vi "Stream_UpdateInfo.vi"(8 "error in (no error)":errorcluster, 9 "Device":string, 10 "SendEventRef":T1, 11 "streams in":variant) -> (0 "error out":errorcluster, 1 "block number":i32, 3 "streams out":variant)   [LabVIEW 2017, in "FileManager.lvlib"]
uses:
  <vilib>/addons/InsightCM/Devices/Shared/Common/FileManager/FileManager.lvlib
  <vilib>/addons/InsightCM/Devices/Shared/Common/FileManager/controls/SendEventRefRoutedMessage.ctl
  <vilib>/addons/InsightCM/Devices/Shared/Common/DataEvent/controls/EventReference.ctl
  <vilib>/addons/InsightCM/Devices/Shared/Common/DataEvent/controls/Event.ctl
  <vilib>/addons/InsightCM/MessageBus/Base/controls/DataEvent.ctl
  <vilib>/addons/InsightCM/MessageBus/Base/controls/KeyValuePair.ctl
  <vilib>/addons/InsightCM/Devices/Shared/Common/DataEvent/controls/DataSet.ctl
  <vilib>/addons/InsightCM/MessageBus/Base/controls/DataSetMetadata.ctl
  <vilib>/addons/InsightCM/MessageBus/Base/controls/TrendPoint.ctl
  <vilib>/addons/InsightCM/MessageBus/Base/controls/TrendAlarmUpdate.ctl
  <vilib>/addons/InsightCM/MessageBus/Base/controls/TrendAlarmTransition.ctl
  <vilib>/addons/InsightCM/Devices/Shared/Common/FileManager/controls/StreamState.ctl
  <vilib>/addons/InsightCM/Devices/Shared/Common/DataEvent/DataEvent.lvlib
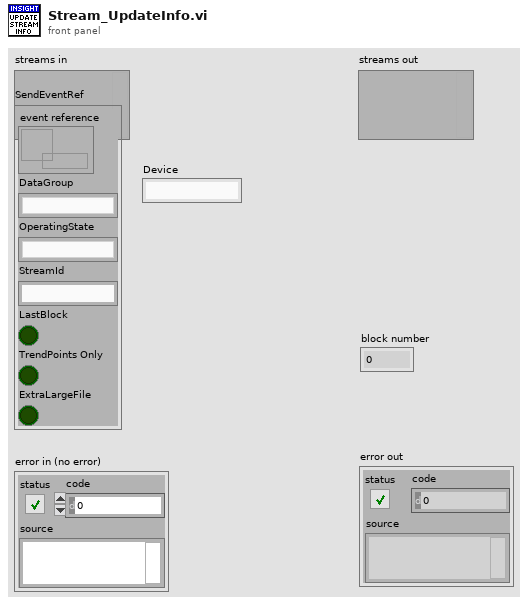
[diagram p1: front panel]
types:
  T1 = typedef "FileManager.lvlib/SendEventRefRoutedMessage.ctl" = cluster{"event reference":T2, "DataGroup":string, "OperatingState":string, "StreamId":string, "LastBlock":bool, "TrendPoints Only":bool, "ExtraLargeFile":bool}
  T2 = typedef "DataEvent.lvlib/EventReference.ctl" = refnum<data-value>
  T3 = typedef "FileManager.lvlib/StreamState.ctl" = cluster{"DataGroup":string, "Stream Id":string, "LastBlock":bool, "TotalBlocks":i32, "BlocksSent":i32, "Device":string}
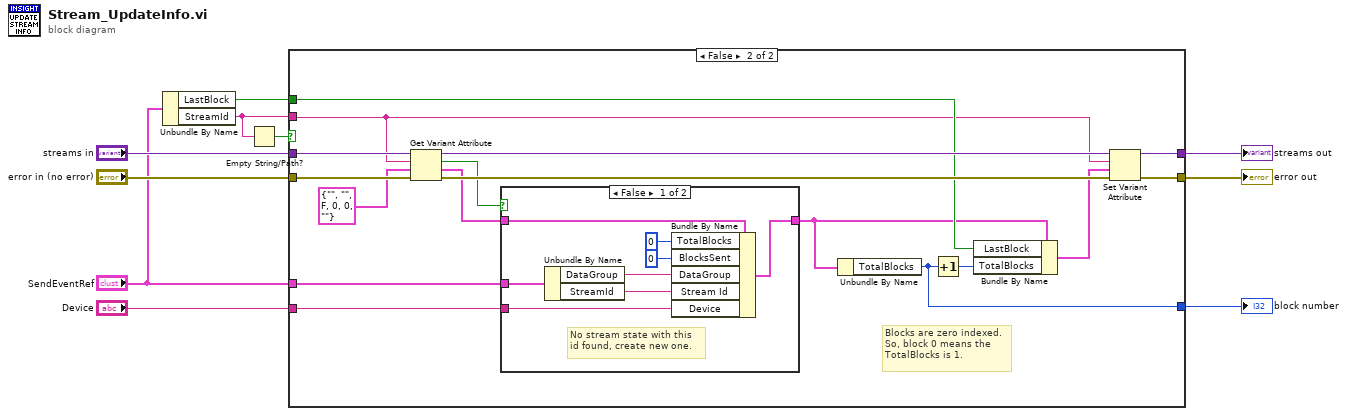
[diagram p0: block diagram]
diagram:
  n1 = Unbundle By Name("SendEventRef") -> ("LastBlock"=w4:bool, "StreamId"=w3:string)
  n2 = Empty String/Path?(string/path=w3) -> (empty?=w2:bool)
  n3 = case shown="False" w2 {
    tunnel: "streams in" -> [w12 w27]
    tunnel: [w12 w26] -> w9
    tunnel: [w11 w25] -> w8
    tunnel: "error in (no error)" -> [w11 w24]
    tunnel: [_ w23] -> w6
    tunnel: "SendEventRef" -> [_ w22]
    tunnel: w4 -> [_ w21]
    tunnel: w3 -> [_ w14]
    tunnel: "Device" -> [_ w13]
    frame True {
      # "If StreamId is empty, this is not a stream"
    }
    frame False {
      # "Blocks are zero indexed.\nSo, block 0 means the\nTotalBlocks is 1."
      n4 = Get Variant Attribute(Variant=w27, name=w14, default value (empty Variant)=T3 {"DataGroup"="", "Stream Id"="", "LastBlock"=FALSE, "TotalBlocks"=0, "BlocksSent"=0, "Device"=""} ("Stream"), error in=w24) -> (duplicate Variant=w28:variant, found=w17:bool, value=w15:T3, error out=w29:errorcluster)
      n5 = case shown="False" w17 {
        tunnel: w15 -> [w34 w38]
        tunnel: w22 -> [w37 _]
        tunnel: [w33 w38] -> w20
        tunnel: w13 -> [w30 _]
        frame False {
          # "No stream state with this \nid found, create new one."
          n6 = Unbundle By Name(w37) -> ("DataGroup"=w32:string, "StreamId"=w31:string)
          n7 = Bundle By Name(cluster=w34, "TotalBlocks"=0, "BlocksSent"=0, "DataGroup"=w32, "Stream Id"=w31, "Device"=w30) -> (w33:T3)
        }
        frame True {
        }
      }
      n8 = Unbundle By Name(w20) -> ("TotalBlocks"=w23:i32)
      n9 = Increment(x=w23) -> (x+1=w19:i32)
      n10 = Bundle By Name(cluster=w20, "LastBlock"=w21, "TotalBlocks"=w19) -> (w18:T3)
      n11 = Set Variant Attribute(Variant=w28, name=w14, value=w18, error in=w29) -> (Variant out=w26:variant, error out=w25:errorcluster)  [unwired: 1 out]
    }
  }
  "streams out" <- w9
  "block number" <- w6
  "error out" <- w8
